vi "MeasureCPU.vi"(8 "error in (no error)":errorcluster, 10 "port number (3363)":u32, 11 "machine name (\"\":  open local reference)":string) -> (0 "error out":errorcluster, 1 "Low Priority":dbl, 2 "Normal Priority":dbl, 3 "High Priority":dbl, 5 "Time Critical":dbl)   [LabVIEW 2010, in "kevLib2010.lvlib"]
uses:
  kevLib2010.lvlib
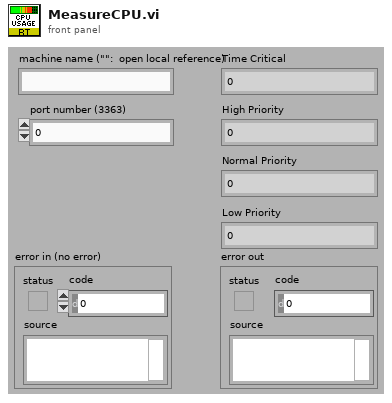
[diagram p1: front panel]
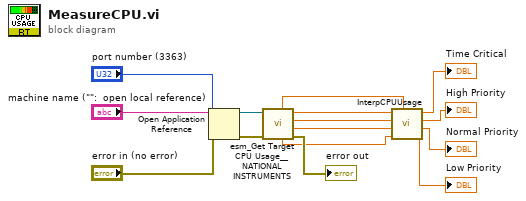
[diagram p0: block diagram]
diagram:
  n1 = Open Application Reference(8:"error in (no error)", 10:"port number (3363)", 11:"machine name (\"\":  open local reference)") -> (0:w15:errorcluster, 3:w14:refnum<vi>)  [unwired: 1 in]
  n2 = call "esm_Get Target CPU Usage__NATIONAL INSTRUMENTS.vi"("error in (no error)"=w15, "application reference"=w14) -> ("error out"=→"error out":errorcluster, "UsageHigh"=w6:dbl, "UsageNormal"=w7:dbl, "UsageLow"=w8:dbl, "UsageTimeCritical"=w5:dbl, "UsageIdle"=w9:dbl)  [unwired: 4 in]
  n3 = call "InterpCPUUsage.vi"("Idle"=w9, "Time Critical"=w5, "High"=w6, "Normal"=w7, "Low"=w8) -> ("Low Priority"=→"Low Priority":dbl, "Normal Priority"=→"Normal Priority":dbl, "High Priority"=→"High Priority":dbl, "Time Critical"=→"Time Critical":dbl)  [unwired: 3 in]
